vi "Init Sim Servo Motor.vi"(8 "error in (no error)":errorcluster, 10 "device ID":T1, 11 "NI_Robotics_Starter Kit Host_Sim_2.0 in":refnum<class "NI_Robotics_Starter Kit Host_Sim_2.0.lvclass">) -> (0 "error out":errorcluster, 3 "NI_Robotics_Starter Kit Host_Sim_2.0 out":refnum<class "NI_Robotics_Starter Kit Host_Sim_2.0.lvclass">)   [LabVIEW 2017, in "NI_Robotics_Starter Kit Host_Sim_2.0.lvclass"]
uses:
  <vilib>/robotics/Starter Kit/2.0/Sim Host Interface/NI_Robotics_Starter Kit Host_Sim_2.0.lvclass
  c:/Program Files (x86)/National Instruments/LabVIEW 2017/vi.lib/robotics/Starter Kit/Host Interface/NI_Robotics_Starter Kit Host.lvclass
  <vilib>/robotics/Simulator/Engine/ctl/DeviceID.ctl
  <vilib>/robotics/Starter Kit/Host Interface/NI_Robotics_Starter Kit Host.lvclass/NI_Robotics_Starter Kit Host.ctl
  <vilib>/robotics/Starter Kit/Servo Motor 2.0/NI_Robotics_Starter Kit Servo Motor_2.0.lvclass
  c:/Program Files (x86)/National Instruments/LabVIEW 2017/vi.lib/robotics/Starter Kit/Servo Motor/NI_Robotics_Starter Kit Servo Motor.lvclass
  <vilib>/robotics/Starter Kit/Host Interface/NI_Robotics_Starter Kit Host.lvclass
  <instrlib>/Hitec HS400 Series/HAIOL/Simulator/Hitec HS400 Series Simulator.lvclass
  <vilib>/robotics/Utilities/NI_Robotics Utilities.lvlib
  <vilib>/robotics/Simulator/NI_Robotics_Simulator.lvlib
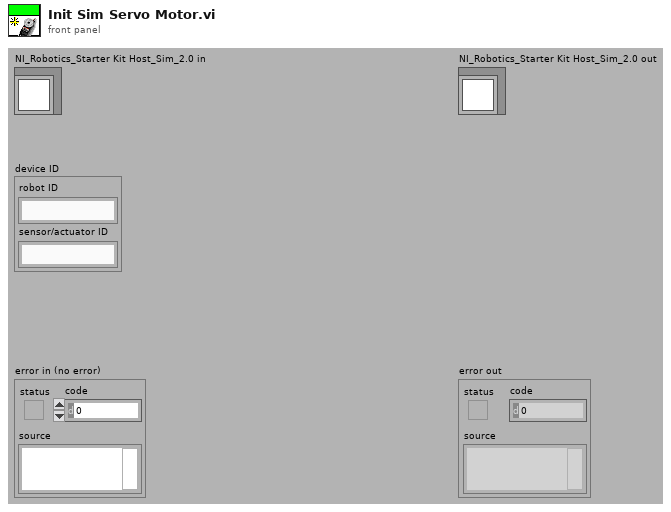
[diagram p1: front panel]
types:
  T1 = typedef "NI_Robotics_Simulator.lvlib/DeviceID.ctl" = cluster{"robot ID":string, "sensor/actuator ID":string}
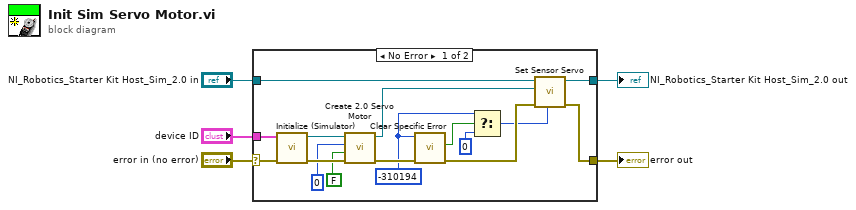
[diagram p0: block diagram]
diagram:
  n1 = case shown="No Error" "error in (no error)" {
    selector: "error in (no error)" -> [w17 w23]
    tunnel: "device ID" -> [w16 _]
    tunnel: "NI_Robotics_Starter Kit Host_Sim_2.0 in" -> [w21 w22]
    tunnel: [w20 w22] -> w1
    tunnel: [w19 w23] -> w2
    frame No Error {
      w8 = -310194 ("code")
      n2 = call <instrlib>:"Initialize (Simulator).vi"("error in (no error)"=w17, "Device ID"=w16) -> ("error out"=w15:errorcluster, "Hitec HS400 Series out"=w14:refnum<class "Hitec HS400 Series.lvclass">)  [unwired: 8 in]
      n3 = call <vilib>:"Create 2.0 Servo Motor.vi"("error in (no error)"=w15, "apply offset angle from file (T)"=FALSE, "servo ID"=0, "Hitec HS400 servo"=w14) -> ("error out"=w11:errorcluster, "Starter Kit Servo Motor_2.0 out"=w18:refnum<class "NI_Robotics_Starter Kit Servo Motor_2.0.lvclass">)  [unwired: 6 in]
      n4 = call <vilib>:"Clear Specific Error.vi"("error in (no error)"=w11, "code"=w8) -> ("error out"=w10:errorcluster, "cleared?"=w9:bool)  [unwired: 7 in, 1 out]
      n5 = Select(t=w8, s=w9, f=0) -> (s? t:f=w6:i32)
      n6 = call <vilib>:"Set Sensor Servo.vi"("sensor servo error (0)"=w6, "error in (no error)"=w10, "sensor servo"=w18, "NI_Robotics_Starter Kit Host in"=w21) -> ("error out"=w19:errorcluster, "NI_Robotics_Starter Kit Host out"=w20:refnum<class "NI_Robotics_Starter Kit Host_Sim_2.0.lvclass">)  [unwired: 6 in]
    }
    frame Error {
    }
  }
  "error out" <- w2
  "NI_Robotics_Starter Kit Host_Sim_2.0 out" <- w1
